vi "Drive_Utils_UpdateState.vi"(0 "delta right":dbl, 1 "delta left":dbl, 2 "speed left":dbl, 3 "speed right":dbl, 4 "error in (no error)":errorcluster) -> (5 "state out":T1, 6 "error out":errorcluster)   [LabVIEW 2009, in "Drive.lvlib" / "Drive_Utils.lvlib"]
uses:
  Drive_Utils.lvlib
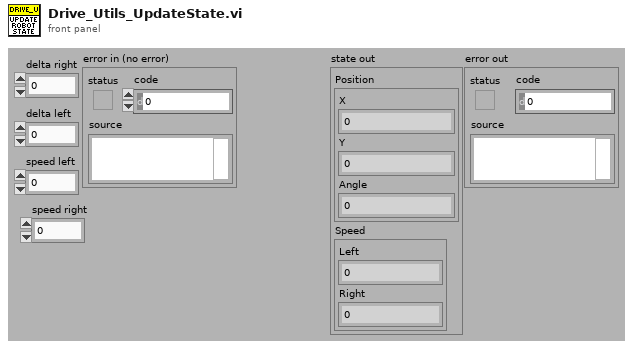
[diagram p1: front panel]
types:
  T1 = cluster{"Position":cluster{"X":dbl, "Y":dbl, "Angle":dbl}, "Speed":cluster{"Left":dbl, "Right":dbl}}
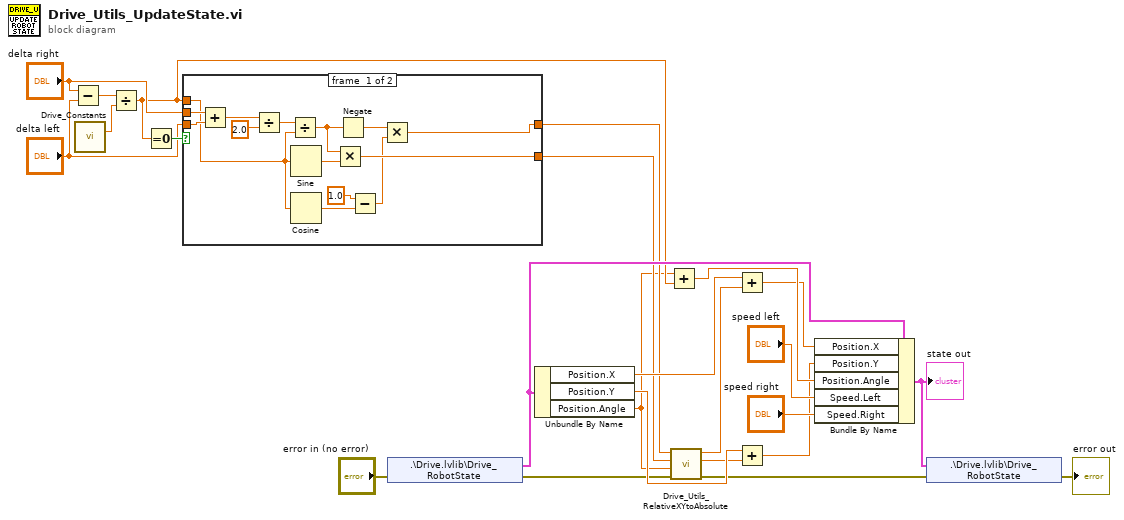
[diagram p0: block diagram]
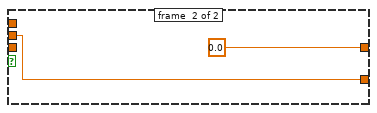
[diagram p2: hidden frame]
diagram:
  n1 = Subtract(x="delta right", y="delta left") -> (x-y=w21:dbl)
  n2 = call "Drive_Constants.vi"() -> ("Wheels interval (m)"=w20:dbl)  [unwired: 23 in, 4 out]
  n3 = Divide(x=w21, y=w20) -> (x/y=w15:dbl)
  n4 = Equal To 0?(x=w15) -> (x = 0?=w18:bool)
  n5 = case shown="False" w18 {
    tunnel: "delta right" -> [w38 w40]
    tunnel: "delta left" -> [w37 _]
    tunnel: w15 -> [w30 _]
    tunnel: [w25 0.0 ("delta right")] -> w7
    tunnel: [w32 w40] -> w6
    frame #0 {
      n6 = Add(x=w38, y=w37) -> (x+y=w36:dbl)
      n7 = Divide(x=w36, y=2.0) -> (x/y=w34:dbl)
      n8 = Divide(x=w34, y=w30) -> (x/y=w31:dbl)
      n9 = Sine(x=w30) -> (sin(x)=w33:dbl)
      n10 = Cosine(x=w30) -> (cos(x)=w29:dbl)
      n11 = Multiply(x=w31, y=w33) -> (x*y=w32:dbl)
      n12 = Negate(x=w31) -> (-x=w27:dbl)
      n13 = Subtract(x=1.0, y=w29) -> (x-y=w26:dbl)
      n14 = Multiply(x=w27, y=w26) -> (x*y=w25:dbl)
    }
    frame #1 {
    }
  }
  n15 = shared-variable ".\\Drive.lvlib\\Drive_RobotState"(error in="error in (no error)") -> (w22:T1, error out=w4:errorcluster)
  n16 = Unbundle By Name(w22) -> ("Position.X"=w14:dbl, "Position.Y"=w12:dbl, "Position.Angle"=w5:dbl)
  n17 = Add(x=w5, y=w15) -> (x+y=w19:dbl)
  n18 = call "Drive_Utils_RelativeXYtoAbsolute.vi"("error in"=w4, "Angle"=w5, "Y"=w6, "X"=w7) -> ("error out"=w3:errorcluster, "Y"=w1:dbl, "X"=w2:dbl)  [unwired: 1 in]
  n19 = Add(x=w14, y=w2) -> (x+y=w13:dbl)
  n20 = Add(x=w12, y=w1) -> (x+y=w11:dbl)
  n21 = Bundle By Name(cluster=w22, "Position.X"=w13, "Position.Y"=w11, "Position.Angle"=w19, "Speed.Left"="speed left", "Speed.Right"="speed right") -> (w10:T1)
  "state out" <- w10
  n22 = shared-variable ".\\Drive.lvlib\\Drive_RobotState"(w10, error in=w3) -> (error out=→"error out":errorcluster)
